vi "DMM_Frequency Domain Meas Configure and Measure.vi"(0 "DMM Handle In":refnum<k15>, 2 "Execution Option":T8, 5 "Function Settings":T6={"Resolution in Digits"=5.5, "Range and Function"=enum."Frequency AC Auto Range"} {"Resolution in Digits" items=["3 1/2"=3.5, "4 1/2"=4.5, "5 1/2"=5.5, "6 1/2"=6.5, "7 1/2"=7.5]}, 7 "Timing & Trigger Settings":T3={"Aperture Time (s)"=-1.0, "Settle Time (s)"=-1.0, "Trigger Settings"={"Trigger Delay (sec)"=-1.0, "Enable Trigger?"=FALSE, "Trigger Source"=enum."Immediate", "Slope"=enum."Rising Edge"}} caption="Timing and Trigger Settings" {"Trigger Settings"."Trigger Delay (sec)" format="%.4f"; "Aperture Time (s)" format="%#.6g"}, 11 "error in":errorcluster) -> (4 "DMM Handle Out":refnum<k15>, 6 "Measurement":T1={"Measured Value"=0.0, "Out of Range"=FALSE, "Unit"="Hertz", "Measurement"="0.0000Hz"} {"Measured Value" format="%^#_9e"}, 8 "DMM Execution Settings":T2={"Absolute\nResolution"=0.0, "Input Resistance\n(Ohm)"=0.0, "Digits\nResolution"=0.0, "Range"=0.0, "Minimum\nFrequency (Hz)"=0.0, "Aperture\nTime (s)"=0.0, "Auto Range\nValue"=0.0, "Settle\nTime (s)"=0.0, "Function"=104} {"Function" items=["DC Volts"=1, "AC Volts"=2, "DC Current"=3, "AC Current"=4, "2-Wire Resistance"=5, "4-Wire Resistance"=101, "Frequency"=104, "Period"=105, "AC Volts DC Coupled"=1001, "Diode"=1002, "Waveform Voltage"=1003, "Waveform Current"=1004, "Capacitance"=1005, "Inductance"=1006, "Temperature"=108]; "Absolute\nResolution" format="%#_6p"; "Input Resistance\n(Ohm)" format="%#_6p"; "Range" format="%#_6p"; "Minimum\nFrequency (Hz)" format="%#_6p"; "Aperture\nTime (s)" format="%#_6p"; "Auto Range\nValue" format="%#_6p"; "Settle\nTime (s)" format="%#_6p"}, 15 "error out":errorcluster)   [LabVIEW 2021, in "DMM_Frequency Domain Measurement.lvlib"]
doc: "Configures an NI-DMM frequency or period measurement on the resource provided by the DMM Handle In control according to the given Function, Execution, and Timing & Trigger settings, and then executes the measurement (by default).\n\nAdditionally users can choose to Configure Only without executing the measurement or Measure Only using the existing configuration."
uses:
  DMM_Frequency Domain Measurement.lvlib
  Common/Typedefs/Execution Options - Measure.ctl
  Typedefs/Function Settings.ctl
  <instrlib>/niDMM/nidmm.llb/niDMM Resolution in Digits.ctl
  Typedefs/Timing & Trigger Settings.ctl
  <instrlib>/niDMM/nidmm.llb/niDMM Trigger.ctl
  <instrlib>/niDMM/nidmm.llb/niDMM Slope.ctl
  Typedefs/DMM Execution Settings.ctl
  Typedefs/Measurement.ctl
  <instrlib>/niDMM/nidmm.llb/niDMM Configure Measurement Digits.vi
panel:
  # "Inputs"
  # "Outputs"
  # "Execution Settings"
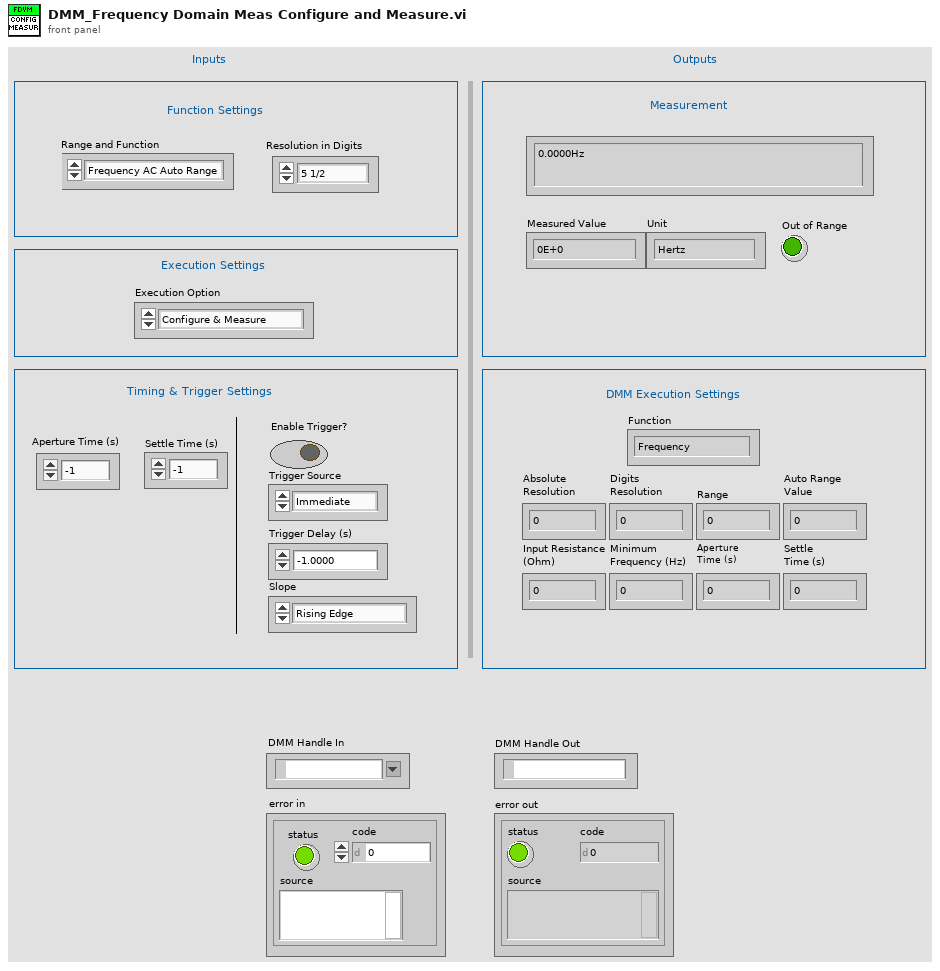
[diagram p1: front panel]
types:
  T1 = typedef "DMM_Frequency Domain Measurement.lvlib/Measurement.ctl" = cluster{"Measured Value":dbl, "Out of Range":bool, "Unit":string, "Measurement":string}
  T2 = typedef "DMM_Frequency Domain Measurement.lvlib/DMM Execution Settings.ctl" = cluster{"Absolute\nResolution":dbl, "Input Resistance\n(Ohm)":dbl, "Digits\nResolution":dbl, "Range":dbl, "Minimum\nFrequency (Hz)":dbl, "Aperture\nTime (s)":dbl, "Auto Range\nValue":dbl, "Settle\nTime (s)":dbl, "Function":i32}
  T3 = typedef "DMM_Frequency Domain Measurement.lvlib/Timing & Trigger Settings.ctl" = cluster{"Aperture Time (s)":dbl, "Settle Time (s)":dbl, "Trigger Settings":cluster{"Trigger Delay (sec)":dbl, "Enable Trigger?":bool, "Trigger Source":T4, "Slope":T5}}
  T4 = typedef "niDMM Trigger.ctl" = enum16{"Immediate", "External", "TTL 0", "TTL 1", "TTL 2", "TTL 3", "TTL 4", "TTL 5", "TTL 6", "Software", "TTL 7", "PXI Star", "LBR Trig 1", "Aux Trig 1"}
  T5 = typedef "niDMM Slope.ctl" = enum16{"Rising Edge", "Falling Edge"}
  T6 = typedef "DMM_Frequency Domain Measurement.lvlib/Function Settings.ctl" = cluster{"Resolution in Digits":T7, "Range and Function":enum16{"Frequency AC Auto Range", "Freq AC 50 mV", "Freq AC 500 mV", "Freq AC 5 V", "Freq AC 50 V", "Freq AC 300 V", "      ", "Period AC Auto Range", "Period AC 50 mV", "Period AC 500 mV", "Period AC 5 V", "Period AC 50 V", "Period AC 300 V"}}
  T7 = typedef "niDMM Resolution in Digits.ctl" = dbl
  T8 = typedef "Execution Options - Measure.ctl" = enum16{"Configure & Measure", "Configure only", "Measure only"}
  T9 = typedef "niDMM Function.ctl" = enum16{"DC Volts", "AC Volts", "DC Current", "AC Current", "2-wire Resistance", "4-wire Resistance", "Diode", "Frequency", "Period", "AC Volts DC Coupled", "Capacitance", "Inductance", "Temperature"}
  T10 = cluster{"Frequency Range":dbl, "Function":T9, "Vertical Range":dbl, "Resolution in Digits":T7}
  T11 = cluster{"Trigger Delay (sec)":dbl, "Enable Trigger?":bool, "Trigger Source":T4, "Slope":T5}
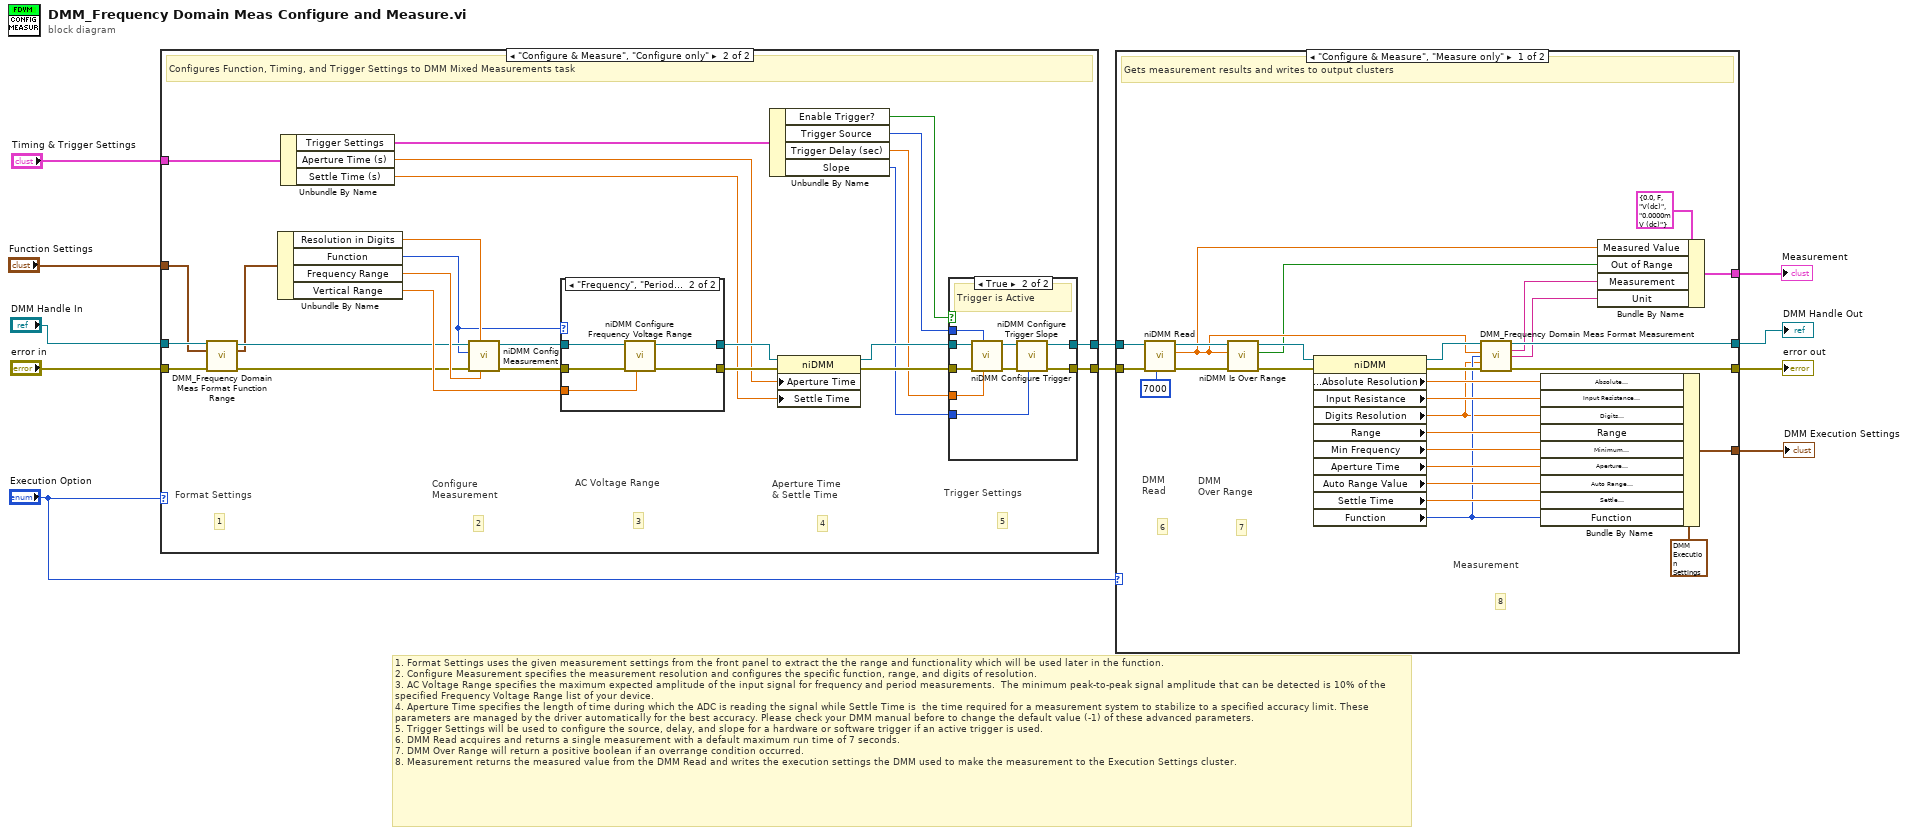
[diagram p0: block diagram]
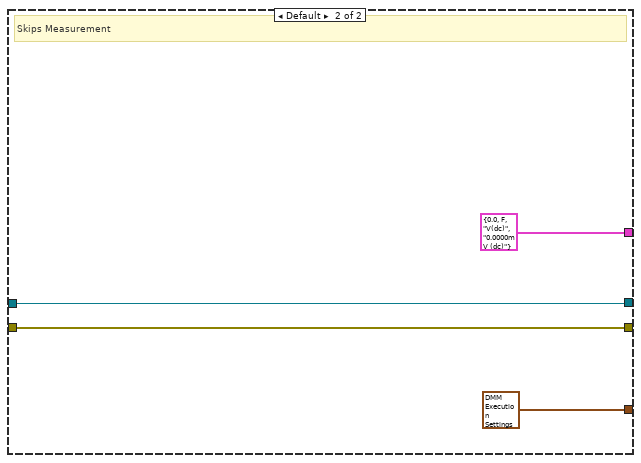
[diagram p2: hidden frame]
diagram:
  # "1. Format Settings uses the given measurement settings from the front panel to extract the the range and functionality which will be used later in the function.\n2. Configure Measurement specifies the measurement resolution and configures the specific function, range, and digits of resolution.\n3. AC Voltage Range specifies the maximum expected amplitude of the input signal for frequency and period measurements.  The minimum peak-to-peak signal amplitude that can be detected is 10% of the specified Frequency Voltage Range list of your device.\n4. Aperture Time specifies the length of time during which the ADC is reading the signal while Settle Time is  the time required for a measurement system to stabilize to a specified accuracy limit. These parameters are managed by the driver automatically for the best accuracy. Please check your DMM manual before to change the default value (-1) of these advanced parameters.\n5. Trigger Settings will be used to configure the source, delay, and slope for a hardware or software trigger if an active trigger is used.\n6. DMM Read acquires and returns a single measurement with a default maximum run time of 7 seconds.\n7. DMM Over Range will return a positive boolean if an overrange condition occurred.\n8. Measurement returns the measured value from the DMM Read and writes the execution settings the DMM used to make the measurement to the Execution Settings cluster."
  n1 = case shown="\"Configure & Measure\", \"Configure only\"" "Execution Option" {
    tunnel: [w13 w37] -> w11
    tunnel: [w12 w36] -> w10
    tunnel: "Timing & Trigger Settings" -> [_ w35]
    tunnel: "DMM Handle In" -> [w13 w20]
    tunnel: "Function Settings" -> [_ w14]
    tunnel: "error in" -> [w12 w18]
    frame "Measure only" {
      # "Skips Configurations (Function, Timing and Trigger Settings)"
    }
    frame "Configure & Measure", "Configure only" {
      # "4"
      # "Aperture Time \n& Settle Time"
      # "1"
      # "Format Settings"
      # "5"
      # "3"
      # "2"
      # "Configure\nMeasurement"
      # "Trigger Settings"
      # "AC Voltage Range"
      # "Configures Function, Timing, and Trigger Settings to DMM Mixed Measurements task"
      n2 = call "DMM_Frequency Domain Meas Format Function Range.vi"("DMM Handle In"=w20, "Function Settings In"=w14, "error in"=w18) -> ("DMM Handle Out"=w19:refnum<k15>, "Function Settings Out"=w16:T10, "error out"=w21:errorcluster)  [unwired: 10 in]
      n3 = Unbundle By Name(w16) -> ("Resolution in Digits"=w17:T7, "Function"=w15:T9, "Frequency Range"=w27:dbl, "Vertical Range"=w25:dbl)
      n4 = Unbundle By Name(w35) -> ("Trigger Settings"=w26:T11, "Aperture Time (s)"=w23:dbl, "Settle Time (s)"=w22:dbl)
      n5 = call-poly <instrlib>:"niDMM Config Measurement.vi"("Range"=w27, "Resolution in Digits"=w17, "error in (no error)"=w21, "Function"=w15, "instrument handle"=w19) -> ("error out"=w32:errorcluster, "instrument handle out"=w34:refnum<k15>)  [unwired: 5 in]
      n6 = case shown="\"Frequency\", \"Period\"" w15 {
        tunnel: w34 -> [w41 w46]
        tunnel: [w41 w45] -> w33
        tunnel: w32 -> [w40 w44]
        tunnel: [w40 w43] -> w31
        tunnel: w25 -> [_ w42]
        frame Default {
        }
        frame "Frequency", "Period" {
          n7 = call <instrlib>:"niDMM Configure Frequency Voltage Range.vi"("Frequency Voltage Range"=w42, "error in (no error)"=w44, "instrument handle"=w46) -> ("error out"=w43:errorcluster, "instrument handle out"=w45:refnum<k15>)  [unwired: 7 in]
        }
      }
      n8 = Unbundle By Name(w26) -> ("Enable Trigger?"=w30:bool, "Trigger Source"=w29:T4, "Trigger Delay (sec)"=w28:dbl, "Slope"=w24:T5)
      n9 = property class="niDMM"(reference=w33, error in=w31, "Aperture Time"=w23, "Settle Time"=w22) -> (reference out=w38:refnum<k15>, error out=w39:errorcluster)
      n10 = case shown="True" w30 {
        tunnel: w39 -> [w47 w56]
        tunnel: w38 -> [w48 w57]
        tunnel: [w48 w51] -> w37
        tunnel: [w47 w50] -> w36
        tunnel: w29 -> [_ w54]
        tunnel: w28 -> [_ w55]
        tunnel: w24 -> [_ w49]
        frame False {
          # "No Trigger"
        }
        frame True {
          # "Trigger is Active"
          n11 = call <instrlib>:"niDMM Configure Trigger.vi"("Trigger Delay (sec)"=w55, "Trigger Source"=w54, "error in (no error)"=w56, "instrument handle"=w57) -> ("error out"=w53:errorcluster, "instrument handle out"=w52:refnum<k15>)  [unwired: 6 in]
          n12 = call <instrlib>:"niDMM Configure Trigger Slope.vi"("Slope"=w49, "error in (no error)"=w53, "instrument handle"=w52) -> ("error out"=w50:errorcluster, "instrument handle out"=w51:refnum<k15>)  [unwired: 7 in]
        }
      }
    }
  }
  n13 = case shown="\"Configure & Measure\", \"Measure only\"" "Execution Option" {
    tunnel: w11 -> [w85 w88]
    tunnel: w10 -> [w84 w89]
    tunnel: [w68 w88] -> w6
    tunnel: [w67 w89] -> w9
    tunnel: [w59 T2 {"Absolute\nResolution"=0.0, "Input Resistance\n(Ohm)"=0.0, "Digits\nResolution"=0.0, "Range"=0.0, "Minimum\nFrequency (Hz)"=0.0, "Aperture\nTime (s)"=0.0, "Auto Range\nValue"=0.0, "Settle\nTime (s)"=0.0, "Function"=1} ("Execution Settings")] -> w2
    tunnel: [w73 T1 {"Measured Value"=0.0, "Out of Range"=FALSE, "Unit"="V(dc)", "Measurement"="0.0000mV (dc)"}] -> w1
    frame "Configure & Measure", "Measure only" {
      # "7"
      # "DMM \nOver Range"
      # "6"
      # "DMM \nRead"
      # "8"
      # "Measurement"
      # "Gets measurement results and writes to output clusters"
      n14 = call <instrlib>:"niDMM Read.vi"("Maximum Time (msec)"=7000, "error in (no error)"=w84, "instrument handle"=w85) -> ("error out"=w82:errorcluster, "Measurement"=w62:dbl, "instrument handle out"=w83:refnum<k15>)  [unwired: 6 in]
      n15 = call <instrlib>:"niDMM Is Over Range.vi"("error in (no error)"=w82, "Measurement"=w62, "instrument handle"=w83) -> ("error out"=w80:errorcluster, "Over Range?"=w61:bool, "instrument handle out"=w81:refnum<k15>)  [unwired: 6 in]
      n16 = property class="niDMM"(reference=w81, error in=w80) -> (reference out=w70:refnum<k15>, error out=w69:errorcluster, "Configuration:Absolute Resolution"=w72:dbl, "Input Resistance"=w79:dbl, "Digits Resolution"=w63:dbl, "Range"=w78:dbl, "Min Frequency"=w77:dbl, "Aperture Time"=w76:dbl, "Auto Range Value"=w75:dbl, "Settle Time"=w74:dbl, "Function"=w64:i32)
      n17 = call "DMM_Frequency Domain Meas Format Measurement.vi"("DMM Handle In"=w70, "Measured Value"=w62, "Function"=w64, "Digits Resolution"=w63, "error in"=w69) -> ("DMM Handle Out"=w68:refnum<k15>, "Measurement"=w66:string, "Unit"=w65:string, "error out"=w67:errorcluster)  [unwired: 7 in]
      n18 = Bundle By Name(cluster=T2 {"Absolute\nResolution"=0.0, "Input Resistance\n(Ohm)"=0.0, "Digits\nResolution"=0.0, "Range"=0.0, "Minimum\nFrequency (Hz)"=0.0, "Aperture\nTime (s)"=0.0, "Auto Range\nValue"=0.0, "Settle\nTime (s)"=0.0, "Function"=1} ("Execution Settings"), "Absolute\nResolution"=w72, "Input Resistance\n(Ohm)"=w79, "Digits\nResolution"=w63, "Range"=w78, "Minimum\nFrequency (Hz)"=w77, "Aperture\nTime (s)"=w76, "Auto Range\nValue"=w75, "Settle\nTime (s)"=w74, "Function"=w64) -> (w59:T2)
      n19 = Bundle By Name(cluster=T1 {"Measured Value"=0.0, "Out of Range"=FALSE, "Unit"="V(dc)", "Measurement"="0.0000mV (dc)"}, "Measured Value"=w62, "Out of Range"=w61, "Measurement"=w66, "Unit"=w65) -> (w73:T1)
    }
    frame Default {
      # "Skips Measurement"
    }
  }
  "error out" <- w9
  "DMM Handle Out" <- w6
  "DMM Execution Settings" <- w2
  "Measurement" <- w1
